vi "Remove response API from List.vi"(10 "API":string, 11 "Output Cluster In":T1[](array[typedef])) -> (3 "Output Cluster Out":T1[](array[typedef]))   [LabVIEW 2017, in "Communicable State Machine.lvlib"]
doc: "### Remove response API from List.vi\n\n-- <b>Controls</b> --\n- <b>API</b>:\n- <b>output cluster in</b>:\n\n-- <b>Indicators</b> --\n- <b>output cluster out</b>:"
uses:
  Communicable State Machine.lvlib
  BroadcastRegistry-Value.ctl
  AdvanceAPI/CSM - Broadcast Message Type.ctl
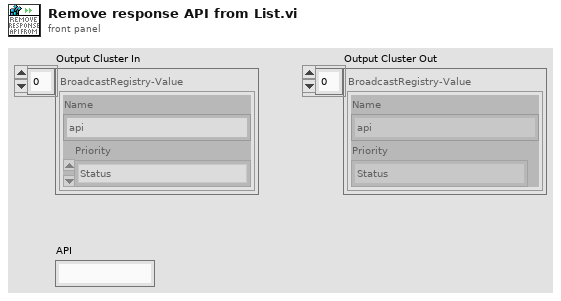
[diagram p1: front panel]
types:
  T1 = typedef "Communicable State Machine.lvlib/BroadcastRegistry-Value.ctl" = cluster{"Name":string, "Priority":T2}
  T2 = typedef "Communicable State Machine.lvlib/CSM - Broadcast Message Type.ctl" = enum16{"Status", "Interrupt"}
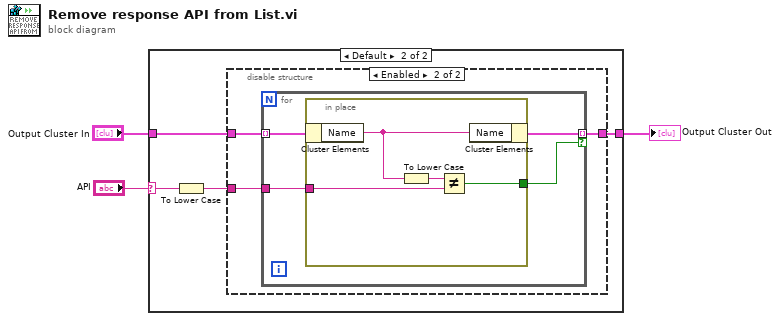
[diagram p0: block diagram]
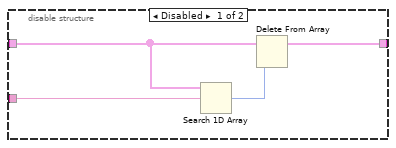
[diagram p3: hidden frame]
diagram:
  n1 = case shown="Default" "API" {
    selector: "API" -> [_ w5]
    tunnel: [_ w7] -> w3
    tunnel: "Output Cluster In" -> [_ w6]
    frame "*" {
    }
    frame Default {
      n2 = To Lower Case(string=w5) -> (all lower case string=w4:string)
      n3 = disable-structure shown="Enabled" {
        disable-tunnel: [w11 w14] -> w7
        disable-tunnel: w6 -> [w10 w13]
        disable-tunnel: w4 -> [w8 w12]
        frame Disabled {
          n4 = Search 1D Array(1D array=w10, element=w8) -> (index of element=w9:i32)  [unwired: 1 in]
          n5 = Delete From Array(array=w10, index=w9) -> (array with subset deleted=w11:T1[])  [unwired: 1 in, 1 out]
        }
        frame Enabled {
          n6 = for {
            tunnel: [w17] -> w14 mode=indexing if=w15
            tunnel: w13 -> [w18] mode=indexing
            tunnel: w12 -> [w16]
            n7 = in-place {
              in-place-border: w16 -> [w21]
              in-place-border: [w19] -> w15
              n8 = in-place-cluster #1(w18) -> ("Name"=w22:string)
              n9 = To Lower Case(string=w22) -> (all lower case string=w20:string)
              n10 = Not Equal?(x=w20, y=w21) -> (x != y?=w19:bool)
              n11 = in-place-cluster #1("Name"=w22) -> (w17:T1)
            }
          }
        }
      }
    }
  }
  "Output Cluster Out" <- w3
